vi "Line Detector Create Regions.vi"(6 "Region width":dbl=500000.0 format="%#_6pHz", 9 "Re-sample":dbl=1.0, 11 "Best fit":dbl[][](array[numeric]) format="%#_4p") -> (3 "Regions frequencies":waveform(dbl)[](array[waveform]))   [LabVIEW 2020]
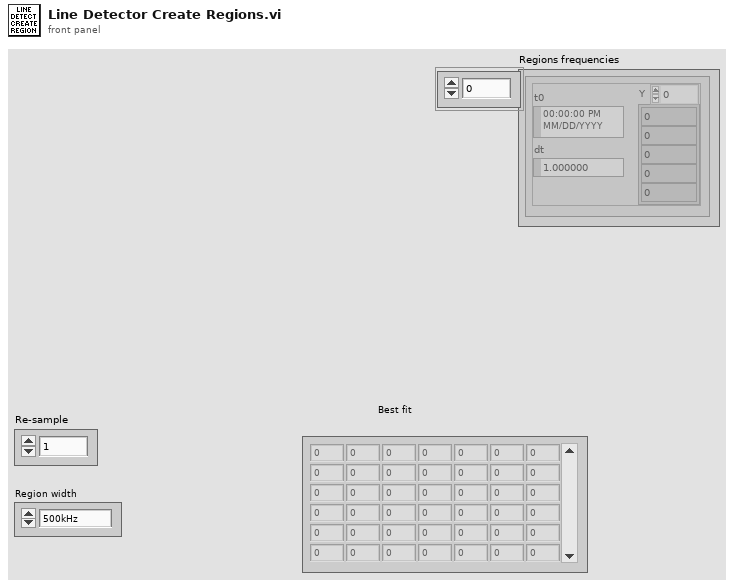
[diagram p1: front panel]
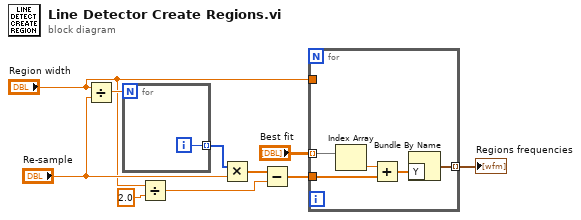
[diagram p0: block diagram]
diagram:
  n1 = Divide(x="Region width", y="Re-sample") -> (x/y=w8:dbl)
  n2 = for {
    N: w8 -> [_]
    tunnel: [w11] -> w7 mode=indexing
    i -> [w11]
  }
  n3 = Divide(x="Region width", y=2.0) -> (x/y=w2:dbl)
  n4 = Multiply(x=w7, y="Re-sample") -> (x*y=w3:dbl[])
  n5 = Subtract(x=w3, y=w2) -> (x-y=w1:dbl[])
  n6 = for {
    tunnel: "Best fit" -> [w16] mode=indexing
    tunnel: "Region width" -> [_]
    tunnel: [w15] -> w9 mode=indexing
    tunnel: w1 -> [w13]
    n7 = Index Array(array=w16) -> (element=w14:dbl)  [unwired: 1 in]
    n8 = Add(x=w14, y=w13) -> (x+y=w12:dbl[])
    n9 = Bundle By Name("Y"=w12) -> (w15:waveform(dbl))  [unwired: 1 in]
  }
  "Regions frequencies" <- w9
